vi "I2CRGBBacklightLCD1602.vi"() -> ()   [LabVIEW 2024]
uses:
  Driver/Public/Digital Pull Direction.ctl
  952d8cb5-7e30-4f7e-8da0-ee00187ed577.vi
  38e447bb-cf5f-4298-9750-7fd1802d0940.vi
  017bc4e3-2c30-43f8-b23f-5495d9bbedc1.vi
  Driver/CTIPicoVISA.lvlib
panel:
  out "Identity":T1
  in  "Grove Connector":enum16{"I2C0", "I2C1"}(ring)
  in  "stop":bool
  in  "Blue":u8(slide) scale=0.0..192.0
  in  "Array":bool[](array[boolean])
  in  "Green":u8(slide) scale=0.0..192.0
  in  "Red":u8(slide) scale=0.0..192.0
  out "blue":u8=250
  out "Green":u8=250
  out "Red":u8=250
  in  "Color Box":u32(colorbox)=16448250
  in  "error in (no error)":errorcluster
  out "error out":errorcluster={"status"=TRUE, "code"=-1073807360, "source"="VISA Write in CTI-Visa.lvlib:Write I2C.vi->RawI2CRGBDemo.vi"}
  in  "Port":refnum<visa-resource-name>="COM7"
  # "Just for Calculating Colours"
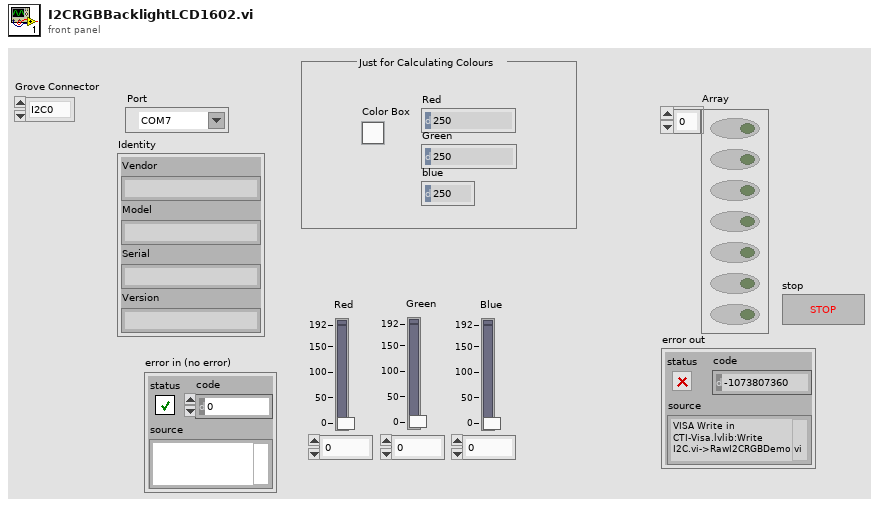
[diagram p1: front panel]
types:
  T1 = cluster{"Vendor":string, "Model":string, "Serial":string, "Version":string}
  T2 = typedef "CTIPicoVISA.lvlib/Digital Pull Direction.ctl" = enum16{"None", "Up", "Down", "Both"}
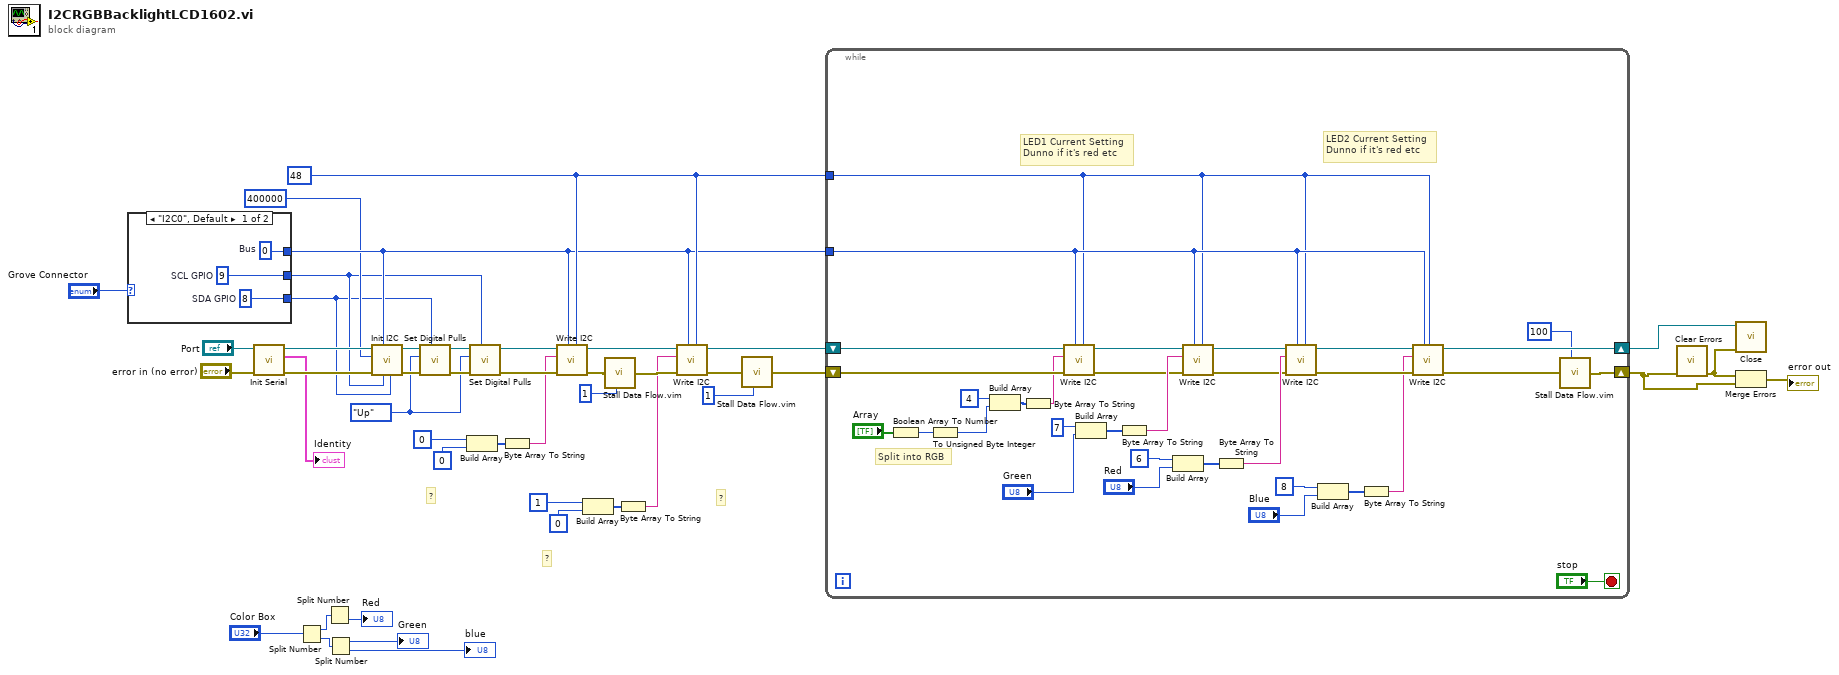
[diagram p0: block diagram]
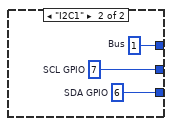
[diagram p2: hidden frame]
diagram:
  w28 = u8 48 ("Address")
  w9 = Digital_Pull_Direction."Up" ("Pull")
  # "?"
  # "?"
  # "?"
  n1 = case shown="\"I2C0\", Default" "Grove Connector" {
    tunnel: [w47 w50] -> w3
    tunnel: [w46 w49] -> w2
    tunnel: [w45 w48] -> w5
    frame "I2C0", Default {
      w45 = u8 0  # Bus
      w46 = 8  # SDA GPIO
      w47 = 9  # SCL GPIO
    }
    frame "I2C1" {
      w48 = u8 1  # Bus
      w49 = 6  # SDA GPIO
      w50 = 7  # SCL GPIO
    }
  }
  n2 = call "Init Serial.vi"("error in (no error)"="error in (no error)", "VISA resource name in"="Port") -> ("error out"=w12:errorcluster, "Identity"=→"Identity":T1, "VISA resource name Out"=w13:refnum<visa-resource-name>)  [unwired: 7 in]
  n3 = Split Number(x="Color Box") -> (hi(x)=w18:u16, lo(x)=w17:u16)
  n4 = Split Number(x=w18) -> (lo(x)=→"Red":u8)  [unwired: 1 out]
  n5 = Split Number(x=w17) -> (hi(x)=→"Green":u8, lo(x)=→"blue":u8)
  n6 = call "Init I2C.vi"("SDA GPIO"=w2, "SCL GPIO"=w3, "Bus"=w5, "error in (no error)"=w12, "Baud"=u32 400000, "VISA resource name in"=w13) -> ("error out"=w43:errorcluster, "VISA resource name"=w42:refnum<visa-resource-name>)  [unwired: 4 in]
  n7 = call "Set Digital Pulls.vi"("GPIO"=w2, "error in (no error)"=w43, "Pull"=w9, "VISA resource name in"=w42) -> ("error out"=w41:errorcluster, "VISA resource name"=w40:refnum<visa-resource-name>)  [unwired: 6 in]
  n8 = Build Array(u8 0 ("Value"), u8 0 ("Value")) -> (w35:u8[])
  n9 = call "Set Digital Pulls.vi"("GPIO"=w3, "error in (no error)"=w41, "Pull"=w9, "VISA resource name in"=w40) -> ("error out"=w37:errorcluster, "VISA resource name"=w38:refnum<visa-resource-name>)  [unwired: 6 in]
  n10 = Byte Array To String(unsigned byte array=w35) -> (string=w34:string)
  n11 = call "Write I2C.vi"("Address"=w28, "Bus"=w5, "error in (no error)"=w37, "Data"=w34, "VISA resource name in"=w38) -> ("error out"=w32:errorcluster, "VISA resource name"=w29:refnum<visa-resource-name>)  [unwired: 5 in]
  n12 = Build Array(u8 1 ("Value"), u8 0 ("Value")) -> (w25:u8[])
  n13 = call "Stall Data Flow.vim"("value in"=w32, "milliseconds to wait"=u32 1) -> ("value out"=w30:errorcluster)  [unwired: 1 out]
  n14 = Byte Array To String(unsigned byte array=w25) -> (string=w23:string)
  n15 = call "Write I2C.vi"("Address"=w28, "Bus"=w5, "error in (no error)"=w30, "Data"=w23, "VISA resource name in"=w29) -> ("error out"=w27:errorcluster, "VISA resource name"=w21:refnum<visa-resource-name>)  [unwired: 5 in]
  n16 = call "Stall Data Flow.vim"("value in"=w27, "milliseconds to wait"=u32 1) -> ("value out"=w20:errorcluster)  [unwired: 1 out]
  n17 = while {
    tunnel: w5 -> [w81]
    tunnel: w28 -> [w80]
    shift-right: [w82] -> w7
    shift-left: w21 -> [w79]
    shift-right: [w83] -> w39
    shift-left: w20 -> [w78]
    stop <- "stop" stop-if-true
    # "LED2 Current Setting\nDunno if it's red etc"
    # "LED1 Current Setting\nDunno if it's red etc"
    # "Split into RGB"
    n18 = Boolean Array To Number(Boolean array="Array") -> (number=w63:u32)
    n19 = To Unsigned Byte Integer(number=w63) -> (unsigned 8bit integer=w62:u8)
    n20 = Build Array(u8 4 ("Value"), w62) -> (w74:u8[])
    n21 = Byte Array To String(unsigned byte array=w74) -> (string=w73:string)
    n22 = call "Write I2C.vi"("Address"=w80, "Bus"=w81, "error in (no error)"=w78, "Data"=w73, "VISA resource name in"=w79) -> ("error out"=w52:errorcluster, "VISA resource name"=w76:refnum<visa-resource-name>)  [unwired: 5 in]
    n23 = Build Array(u8 7 ("GreenAddr"), "Green") -> (w71:u8[])
    n24 = Byte Array To String(unsigned byte array=w71) -> (string=w70:string)
    n25 = Build Array(u8 6 ("Value"), "Red") -> (w68:u8[])
    n26 = call "Write I2C.vi"("Address"=w80, "Bus"=w81, "error in (no error)"=w52, "Data"=w70, "VISA resource name in"=w76) -> ("error out"=w53:errorcluster, "VISA resource name"=w75:refnum<visa-resource-name>)  [unwired: 5 in]
    n27 = Byte Array To String(unsigned byte array=w68) -> (string=w67:string)
    n28 = call "Write I2C.vi"("Address"=w80, "Bus"=w81, "error in (no error)"=w53, "Data"=w67, "VISA resource name in"=w75) -> ("error out"=w60:errorcluster, "VISA resource name"=w59:refnum<visa-resource-name>)  [unwired: 5 in]
    n29 = Build Array(u8 8 ("Value"), "Blue") -> (w57:u8[])
    n30 = Byte Array To String(unsigned byte array=w57) -> (string=w55:string)
    n31 = call "Write I2C.vi"("Address"=w80, "Bus"=w81, "error in (no error)"=w60, "Data"=w55, "VISA resource name in"=w59) -> ("error out"=w54:errorcluster, "VISA resource name"=w82:refnum<visa-resource-name>)  [unwired: 5 in]
    n32 = call "Stall Data Flow.vim"("value in"=w54, "milliseconds to wait"=u32 100) -> ("value out"=w83:errorcluster)  [unwired: 1 out]
  }
  n33 = call <vilib>:"Clear Errors.vi"("error in (no error)"=w39) -> ("error out"=w8:errorcluster)  [unwired: 5 in, 1 out]
  n34 = call "Close.vi"("error in (no error)"=w8, "VISA resource name in"=w7) -> ()  [unwired: 9 in, 1 out]
  n35 = Merge Errors(w8, w39) -> (→"error out":errorcluster)
